vi "Inject Fan Controller.vi"(8 "error in (no error)":errorcluster, 10 "Fan Controller Ref":refnum<data-value>, 11 "Process Model in":refnum<class "Process Model.lvclass">) -> (0 "error out":errorcluster, 3 "Process Model out":refnum<class "Process Model.lvclass">)   [LabVIEW 2019, in "Process Model.lvclass"]
uses:
  <vilib>/gpm_packages/@cs/Car-wash/Source/Process Model/Process Model.lvclass
  <vilib>/gpm_packages/@cs/Car-wash/Source/iFan Controller/iFan Controller.lvclass
  <vilib>/gpm_packages/@cs/Car-wash/Source/Process Model/Process Model.lvclass/Process Model.ctl
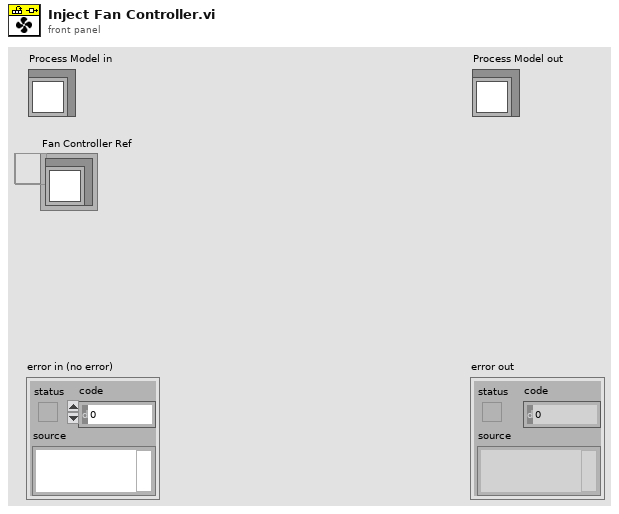
[diagram p1: front panel]
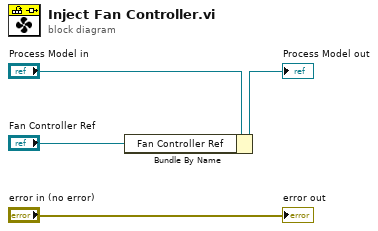
[diagram p0: block diagram]
diagram:
  n1 = Bundle By Name(cluster="Process Model in", "Fan Controller Ref"="Fan Controller Ref") -> (→"Process Model out":refnum<class "Process Model.lvclass">)
  "error out" <- "error in (no error)"
